vi "Robot Global Data.vi"() -> ()   [LabVIEW 2017]
doc: "This global VI can contain as many global variables as you need. Place a control on the panel, give it a good name. To read or write to it from a VI, drag the icon to the diagram of that VI. You can also drag from the project. Click on the node to change which global you access. You shouldn't have multiple locations writing to a global or it will cause a race-condition."
uses:
  <vilib>/Rock Robotics/WPI/Camera/WPI_CameraImageSize.ctl
  <vilib>/Rock Robotics/WPI/DriverStation/WPI_DriverStationRobotMode2.ctl
  Lift States.ctl
panel:
  out "Robot Disabled?":bool
  out "Lift Moving":bool
  out "Intake Suck In":bool
  out "Intake Spit Out":bool
  out "Got the Loot":bool=TRUE
  out "At Lift Setpoint?":bool
  out "Lift Stop":bool
  in  "Lift HODL Setpoint":dbl
  in  "Lift Setpoint":dbl
  in  "Intake Speed":dbl
  out "Intake Angle Down":bool
  out "Intake Arms In":bool=TRUE
  out "Engage Low Gear":bool
  in  "Auto Selector":string
  out "AUTO Switch Scale Mismatch":bool
  out "AUTO Scale Right":bool
  out "AUTO Switch Right":bool
  out "AUTO Start Left":bool
  out "Manual Lift Speed":dbl
  out "Lift Position":dbl
  out "Lift State":T1
  out "Zero Drive Encoder?":bool
  in  "Drive Encoder Offset":dbl
  out "Drive Encoder":dbl
  in  "Right Drive Speed":dbl min=-1.0 max=1.0
  in  "Left Drive Speed":dbl min=-1.0 max=1.0
  out "Zero Heading?":bool
  in  "Heading Offset":dbl
  out "Current Heading":dbl
  in  "Robot Mode":T2
  in  "image size":T3=enum."320x240"
  in  "Enable Vision":bool
  # "RED"
  # "Left Side Reverse #1 turns"
  # "Mismatch Reverse #2 turns"
  # "YELLOW"
  # "GREEN"
  # "BLUE"
  # "WHITE"
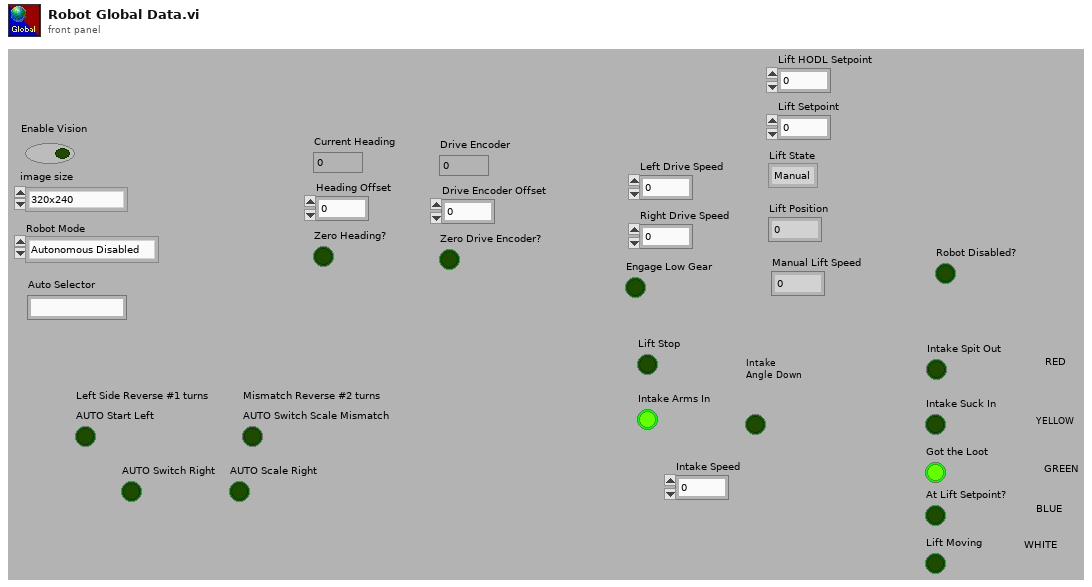
[diagram p1: front panel]
types:
  T1 = typedef "Lift States.ctl" = enum16{"Manual", "Scale Low", "Scale Middle", "Scale High", "Rock Bottom", "Almost Down"}
  T2 = typedef "WPI_DriverStationRobotMode2.ctl" = enum16{"Autonomous Disabled", "Autonomous Enabled", "Teleop Disabled", "Teleop Enabled", "Disconnected", "Finish", "Test Disabled", "Test Enabled", "Emergency Stopped"}
  T3 = typedef "WPI_CameraImageSize.ctl" = enum16{"640x480", "320x240", "160x120", "Custom"}
diagram:
